vi "F.C.C (SubVI).vi"(6 "Tm":dbl, 9 "THETA":dbl, 10 "TAO":dbl, 11 "K":dbl) -> (1 "Numeric":dbl, 2 "Numeric 2":dbl, 3 "Numeric 3":dbl)   [LabVIEW 2020]
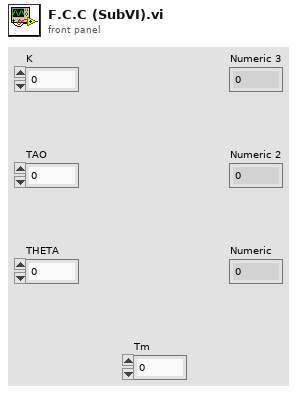
[diagram p1: front panel]
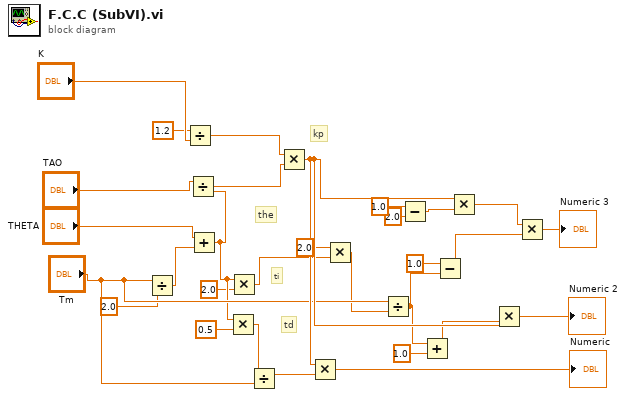
[diagram p0: block diagram]
diagram:
  # "td"
  # "ti"
  # "the"
  # "kp"
  n1 = Divide(x="Tm", y=2.0) -> (x/y=w2:dbl)
  n2 = Divide(x=1.2, y="K") -> (x/y=w7:dbl)
  n3 = Add(x="THETA", y=w2) -> (x+y=w10:dbl)
  n4 = Divide(x="TAO", y=w10) -> (x/y=w8:dbl)
  n5 = Multiply(x=w10, y=0.5) -> (x*y=w26:dbl)
  n6 = Multiply(x=w10, y=2.0) -> (x*y=w12:dbl)
  n7 = Divide(x=w26, y="Tm") -> (x/y=w28:dbl)
  n8 = Multiply(x=w7, y=w8) -> (x*y=w29:dbl)
  n9 = Multiply(x=w29, y=w28) -> (x*y=→"Numeric":dbl)
  n10 = Multiply(x=2.0, y=w12) -> (x*y=w14:dbl)
  n11 = Divide(x="Tm", y=w14) -> (x/y=w19:dbl)
  n12 = Subtract(x=1.0, y=2.0) -> (x-y=w21:dbl)
  n13 = Add(x=w19, y=1.0) -> (x+y=w16:dbl)
  n14 = Subtract(x=1.0, y=w19) -> (x-y=w23:dbl)
  n15 = Multiply(x=w29, y=w21) -> (x*y=w22:dbl)
  n16 = Multiply(x=w29, y=w16) -> (x*y=→"Numeric 2":dbl)
  n17 = Multiply(x=w22, y=w23) -> (x*y=→"Numeric 3":dbl)
